vi "test_Series cRIO PWM CAN Temp.vi"(8 "Error In":errorcluster) -> (0 "Error Out":errorcluster)   [LabVIEW 2023]
uses:
  Series/Series Base/Series Base.lvclass
  Series/Series Actor/Series Actor/Series Actor.lvclass
  DIO/DO DAQmx Fixed Freq PWM CFG/DO DAQmx Fixed Freq PWM CFG.lvclass
  Sample Tasks/Sample Temp PWM Control/Sample Temp PWM Control.lvclass
  Devices/NEO480HTA/Real All CFG/Read All CFG.lvclass
  DIO/Virtual DIO/Virt PWM Fixed Freq Generator/Virt PWM Fixed Freq Generator.lvclass
  Series/Series Base/Series Base.lvclass/Series Base.ctl
  Task/Task Base/Task Base.lvclass/Task Base.ctl
  Series/Series Actor/Series Actor/Series Actor.lvclass/Series Actor.ctl
  <vilib>/ActorFramework/Message Enqueuer/Message Enqueuer.lvclass/Message Enqueuer.ctl
  <vilib>/ActorFramework/Stop Msg/Stop Msg.lvclass/Stop Msg.ctl
  Series/Series Base/Get Task.vi
  <vilib>/ActorFramework/Message Enqueuer/Enqueue.vi
  <vilib>/ActorFramework/Message Enqueuer/Enqueue Critical.vi
  Series/ISeries Actor/ISeries Actor Messages/Stop Tasks Msg/Stop Tasks Msg.lvclass
  <vilib>/ActorFramework/Stop Msg/Stop Msg.lvclass
  <vilib>/Utility/error.llb/Error Cluster From Error Code.vi
  <vilib>/Utility/LVClass/Get LV Class Name.vi
  <resource>/AFDebug/Generate Trace for Message.vi
  <vilib>/ActorFramework/Message Priority Queue/Priority Enqueue.vi
  <vilib>/ActorFramework/Actor/Actor.lvclass
  Series/ISeries Actor/ISeries Actor Messages/Start Tasks Msg/Start Tasks Msg.lvclass
  C:/Program Files/National Instruments/LabVIEW 2023/vi.lib/ActorFramework/Actor/Actor.lvclass
  D:/git/HAL/HAL GOOP4/Series/Series Actor/Series Actor/Series Actor.lvclass
  D:/git/HAL/HAL GOOP4/Series/ISeries Actor/ISeries Actor/ISeries Actor.lvclass
panel:
  in  "Start Series Button":bool
  in  "Kill Series Actor Button":bool
  out "Temperature Chart Lossy":dbl(graph)
  in  "Temp Setpoint":dbl=23.0 format="%#_g °C"
  in  "stop":bool
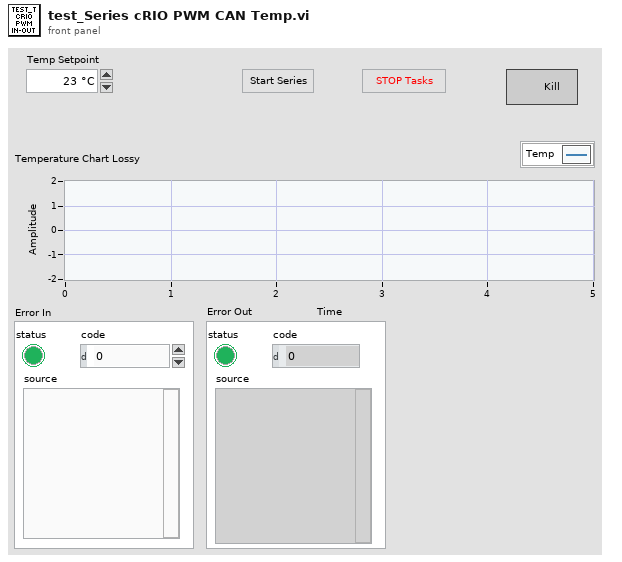
[diagram p1: front panel]
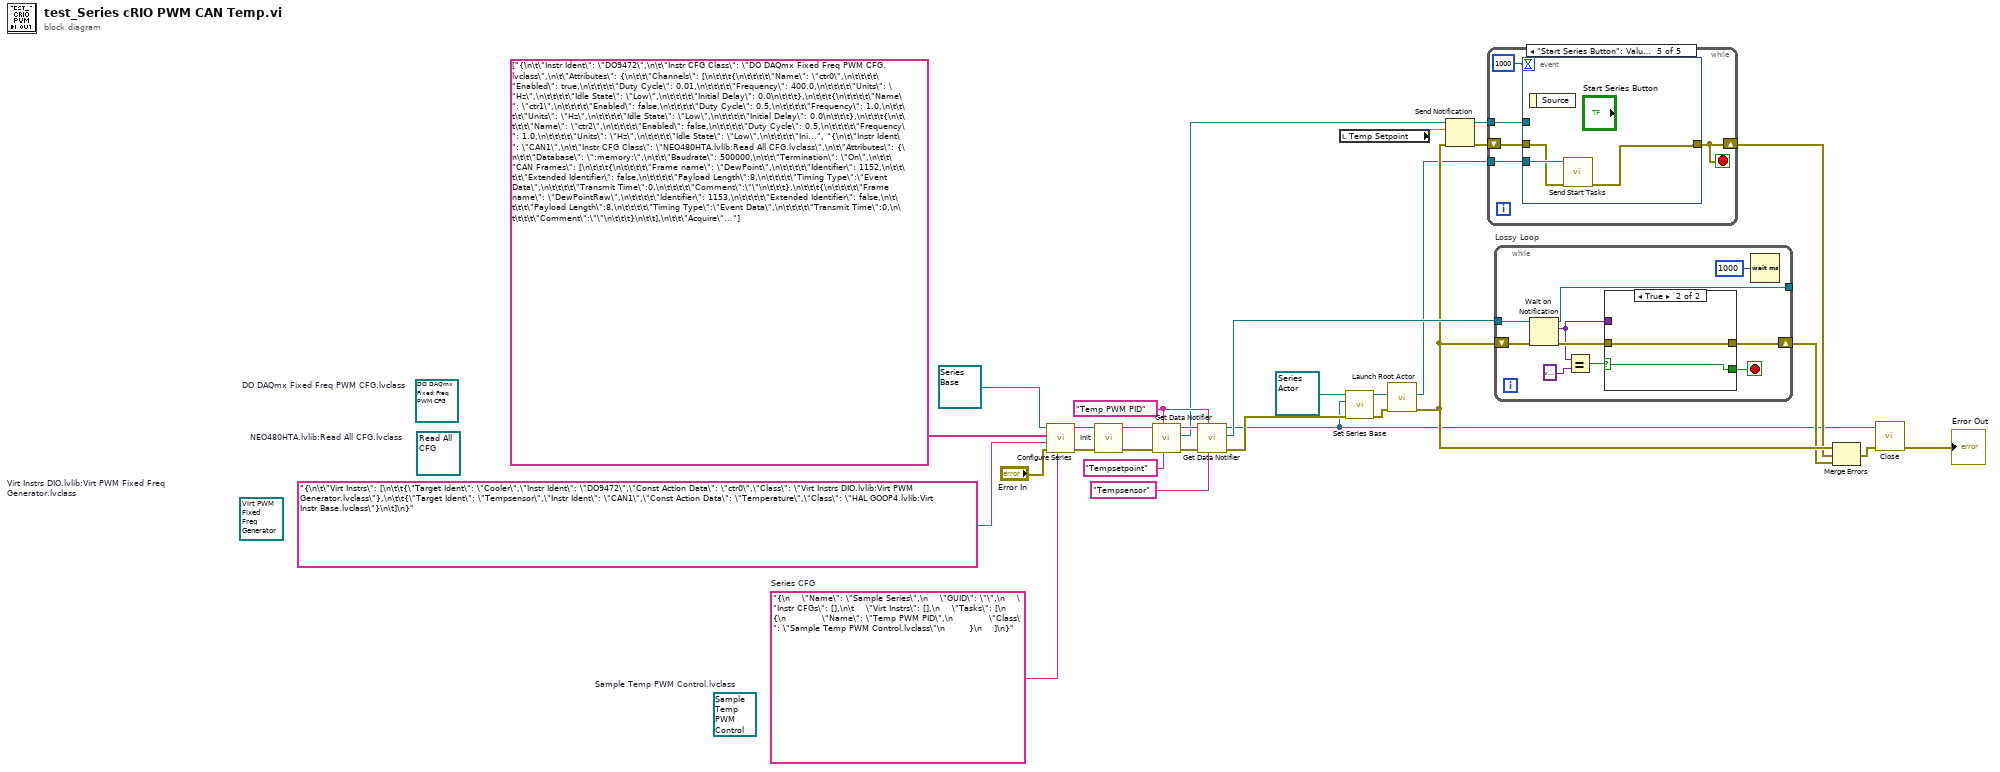
[diagram p0: block diagram]
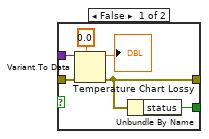
[diagram p2: hidden frame]
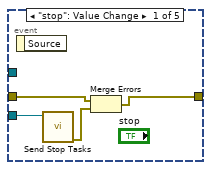
[diagram p3: hidden frame]
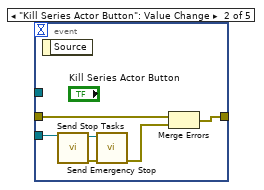
[diagram p4: hidden frame]
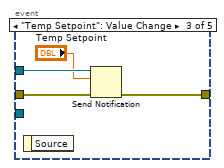
[diagram p5: hidden frame]
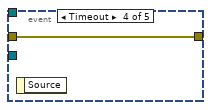
[diagram p6: hidden frame]
diagram:
  w10 = "Temp PWM PID"
  (unwired) refnum<class "Virt PWM Fixed Freq Generator.lvclass"> refnum  # Virt Instrs DIO.lvlib:Virt PWM Fixed Freq Generator.lvclass
  w27 = "{\n    \"Name\": \"Sample Series\",\n    \"GUID\": \"\",\n    \"Instr CFGs\": [],\n\t    \"Virt Instrs\": [],\n    \"Tasks\": [\n        {\n            \"Name\": \"Temp PWM PID\",\n            \"Class\": \"Sample Temp PWM Control.lvclass\"\n        }\n    ]\n}"  # Series CFG
  (unwired) refnum<class "Read All CFG.lvclass"> refnum  # NEO480HTA.lvlib:Read All CFG.lvclass
  (unwired) refnum<class "Sample Temp PWM Control.lvclass"> refnum  # Sample Temp PWM Control.lvclass
  (unwired) refnum<class "DO DAQmx Fixed Freq PWM CFG.lvclass"> refnum  # DO DAQmx Fixed Freq PWM CFG.lvclass
  n1 = call "Configure Series.vi"("Series CFG"=w27, "error in (no error)"="Error In", "Virt Instrs CFG"="{\n\t\"Virt Instrs\": [\n\t\t{\"Target Ident\": \"Cooler\",\"Instr Ident\": \"DO9472\",\"Const Action Data\": \"ctr0\",\"Class\": \"Virt Instrs DIO.lvlib:Virt PWM Generator.lvclass\"},\n\t\t{\"Target Ident\": \"Tempsensor\",\"Instr Ident\": \"CAN1\",\"Const Action Data\": \"Temperature\",\"Class\": \"HAL GOOP4.lvlib:Virt Instr Base.lvclass\"}\n\t]\n}", "Instr CFGs"=string[] ["{\n\t\"Instr Ident\": \"DO9472\",\n\t\"Instr CFG Class\": \"DO DAQmx Fixed Freq PWM CFG.lvclass\",\n\t\"Attributes\": {\n\t\t\"Channels\": [\n\t\t\t{\n\t\t\t\t\"Name\": \"ctr0\",\n\t\t\t\t\"Enabled\": true,\n\t\t\t\t\"Duty Cycle\": 0.01,\n\t\t\t\t\"Frequency\": 400.0,\n\t\t\t\t\"Units\": \"Hz\",\n\t\t\t\t\"Idle State\": \"Low\",\n\t\t\t\t\"Initial Delay\": 0.0\n\t\t\t},\n\t\t\t{\n\t\t\t\t\"Name\": \"ctr1\",\n\t\t\t\t\"Enabled\": false,\n\t\t\t\t\"Duty Cycle\": 0.5,\n\t\t\t\t\"Frequency\": 1.0,\n\t\t\t\t\"Units\": \"Hz\",\n\t\t\t\t\"Idle State\": \"Low\",\n\t\t\t\t\"Initial Delay\": 0.0\n\t\t\t},\n\t\t\t{\n\t\t\t\t\"Name\": \"ctr2\",\n\t\t\t\t\"Enabled\": false,\n\t\t\t\t\"Duty Cycle\": 0.5,\n\t\t\t\t\"Frequency\": 1.0,\n\t\t\t\t\"Units\": \"Hz\",\n\t\t\t\t\"Idle State\": \"Low\",\n\t\t\t\t\"Initial Delay\": 0.0\n\t\t\t},\n\t\t\t{\n\t\t\t\t\"Name\": \"ctr3\",\n\t\t\t\t\"Enabled\": false,\n\t\t\t\t\"Duty Cycle\": 0.5,\n\t\t\t\t\"Frequency\": 1.0,\n\t\t\t\t\"Units\": \"Hz\",\n\t\t\t\t\"Idle State\": \"Low\",\n\t\t\t\t\"Initial Delay\": 0.0\n\t\t\t}\n\t\t],\n\t\t\"Timing\": {\n\t\t\t\"Samples per Channel\": 1000,\n\t\t\t\"Sample Mode\": \"Continuous Samples\",\n\t\t\t\"Sample Rate\": 0.0,\n\t\t\t\"Sample Clock Source\": \"Implicit\",\n\t\t\t\"Active Edge\": \"Rising\"\n\t\t},\n\t\t\"Trigger\": {\n\t\t\t\"Trigger Type\": \"No Trigger\"\n\t\t}\n\t}\n}", "{\n\t\"Instr Ident\": \"CAN1\",\n\t\"Instr CFG Class\": \"NEO480HTA.lvlib:Read All CFG.lvclass\",\n\t\"Attributes\": {\n\t\t\"Database\": \":memory:\",\n\t\t\"Baudrate\": 500000,\n\t\t\"Termination\": \"On\",\n\t\t\"CAN Frames\": [\n\t\t\t{\n\t\t\t\t\"Frame name\": \"DewPoint\",\n\t\t\t\t\"Identifier\": 1152,\n\t\t\t\t\"Extended Identifier\": false,\n\t\t\t\t\"Payload Length\":8,\n\t\t\t\t\"Timing Type\":\"Event Data\",\n\t\t\t\t\"Transmit Time\":0,\n\t\t\t\t\"Comment\":\"\"\n\t\t\t},\n\t\t\t{\n\t\t\t\t\"Frame name\": \"DewPointRaw\",\n\t\t\t\t\"Identifier\": 1153,\n\t\t\t\t\"Extended Identifier\": false,\n\t\t\t\t\"Payload Length\":8,\n\t\t\t\t\"Timing Type\":\"Event Data\",\n\t\t\t\t\"Transmit Time\":0,\n\t\t\t\t\"Comment\":\"\"\n\t\t\t}\n\t\t],\n\t\t\"Acquire\": {\n\t\t\t\"Type\": \"Read Frame\"\n\t\t}\n\t}\n}"], "HAL GOOP4:Series Base in"=refnum<class "Series Base.lvclass"> refnum ("HAL GOOP4.lvlib:Study Base.lvclass")) -> ("error out"=w29:errorcluster, "HAL GOOP4:Series Base out"=w30:refnum<class "Series Base.lvclass">)  [unwired: 5 in]
  n2 = call-dynamic "Init.vi"("error in (no error)"=w29, "HAL GOOP4:Series Base in"=w30) -> ("error out"=w23:errorcluster, "HAL GOOP4:Series Base out"=w18:refnum<class "Series Base.lvclass">)  [unwired: 8 in]
  n3 = call "Get Data Notifier.vi"("Notifier Name"="Tempsetpoint" ("Name"), "Task Name"=w10, "error in (no error)"=w23, "Series Base in"=w18) -> ("error out"=w19:errorcluster, "Data Notifier"=w6:refnum<notifier>, "Series Base out"=w12:refnum<class "Series Base.lvclass">)  [unwired: 5 in]
  n4 = call "Get Data Notifier.vi"("Notifier Name"="Tempsensor" ("Target Name"), "Task Name"=w10, "error in (no error)"=w19, "Series Base in"=w12) -> ("error out"=w13:errorcluster, "Data Notifier"=w9:refnum<notifier>, "Series Base out"=w1:refnum<class "Series Base.lvclass">)  [unwired: 5 in]
  n5 = local read "Temp Setpoint"() -> (w20:dbl)
  n6 = call "Set Series Base.vi"("error in (no error)"=w13, "Series Base"=w1, "Series Actor in"=refnum<class "Series Actor.lvclass"> refnum ("Series Actor.lvlib:Series Actor.lvclass")) -> ("error out"=w17:errorcluster, "Series Actor out"=w16:refnum<class "Series Actor.lvclass">)  [unwired: 7 in]
  n7 = call <vilib>:"Launch Root Actor.vi"("error in (no error)"=w17, "Actor"=w16) -> ("error out"=w8:errorcluster, "Actor's Enqueuer"=w7:refnum<class "Message Enqueuer.lvclass">)  [unwired: 8 in]
  n8 = Send Notification(notification=w20, notifier=w6, error in (no error)=w8) -> (notifier out=w5:refnum<notifier>, error out=w21:errorcluster)
  n9 = while {
    shift-right: [w35] -> w2
    shift-left: w21 -> [w34]
    tunnel: w7 -> [w33]
    tunnel: w5 -> [w32]
    stop <- w35 stop-if-true
    n10 = event shown="[4] \"Start Series Button\": Value Change" {
      selector: _ -> [_ _ _ _ _]
      dyn-events: _ -> [_ _ _ _ _]
      timeout: 1000 -> [_ _ _ _ _]
      tunnel: [w36 w43 w47 w50 w51] -> w35
      tunnel: w32 -> [_ _ w49 _ _]
      tunnel: w34 -> [w37 w42 w46 w50 w52]
      tunnel: w33 -> [w39 w45 _ _ w53]
      event "stop": Value Change {
        n11 = event-data() -> ()  [unwired: 1 in, 1 out]
        n12 = call "Send Stop Tasks.vi"("Message Enqueuer"=w39) -> ("error out"=w38:errorcluster)  [unwired: 9 in, 1 out]
        n13 = Merge Errors(w37, w38) -> (w36:errorcluster)
      }
      event "Kill Series Actor Button": Value Change {
        n14 = event-data() -> ()  [unwired: 1 in, 1 out]
        n15 = call "Send Stop Tasks.vi"("Message Enqueuer"=w45) -> ("error out"=w44:errorcluster, "Message Enqueuer out"=w40:refnum<class "Message Enqueuer.lvclass">)  [unwired: 9 in]
        n16 = call <vilib>:"Send Emergency Stop.vi"("error in (no error)"=w44, "Message Enqueuer"=w40) -> ("error out"=w41:errorcluster)  [unwired: 9 in]
        n17 = Merge Errors(w42, w41) -> (w43:errorcluster)
      }
      event "Temp Setpoint": Value Change {
        n18 = event-data() -> ()  [unwired: 1 in, 1 out]
        n19 = Send Notification(notification="Temp Setpoint", notifier=w49, error in (no error)=w46) -> (error out=w47:errorcluster)  [unwired: 1 out]
      }
      event Timeout {
        n20 = event-data() -> ()  [unwired: 1 in, 1 out]
      }
      event "Start Series Button": Value Change {
        n21 = event-data() -> ()  [unwired: 1 in, 1 out]
        n22 = call "Send Start Tasks.vi"("error in (no error)"=w52, "Message Enqueuer"=w53) -> ("error out"=w51:errorcluster)  [unwired: 8 in, 1 out]
      }
    }
  }
  n23 = while "Lossy Loop" {
    tunnel: w9 -> [w59]
    shift-right: [w60] -> w3
    shift-left: w8 -> [w61]
    tunnel: [w58] -> _
    stop <- w57 stop-if-true
    n24 = Wait on Notification(notifier=w59, error in (no error)=w61) -> (notifier out=w58:refnum<notifier>, notification=w55:variant, error out=w63:errorcluster)  [unwired: 2 in, 1 out]
    n25 = Equal?(x=w55, y=variant) -> (x = y?=w54:bool)
    n26 = case shown="True" w54 {
      selector: w54 -> [_ w71]
      tunnel: w63 -> [w69 w70]
      tunnel: [w67 w70] -> w60
      tunnel: [w64 w71] -> w57
      tunnel: w55 -> [w65 _]
      frame False {
        n27 = Variant To Data(error in=w69, type=0.0 ("Waveform"), Variant=w65) -> (data=→"Temperature Chart Lossy":dbl, error out=w67:errorcluster)
        n28 = Unbundle By Name(w67) -> ("status"=w64:bool)
      }
      frame True {
      }
    }
    n29 = Wait (ms)(milliseconds to wait=u32 1000) -> ()  [unwired: 1 out]
  }
  n30 = Merge Errors(w8, w2, w3) -> (w4:errorcluster)
  n31 = call-dynamic "Close.vi"("error in (no error)"=w4, "HAL GOOP4:Series Base in"=w1) -> ("error out"=→"Error Out":errorcluster)  [unwired: 8 in, 1 out]
